vi "Quit.vi"(8 "error in (no error)":errorcluster, 11 "Axis in":refnum<class "Axis.lvclass">) -> (0 "error out":errorcluster)   [LabVIEW 2020, in "Axis.lvclass"]
uses:
  Axis.lvclass
  C:/Users/Jonathan/Documents/Clearpath SDK/CSharp Examples/CLRWrapper/x64/Debug/CLRWrapper.dll
  CSharp Examples/CLRWrapper/x64/Debug/CLRWrapper.dll
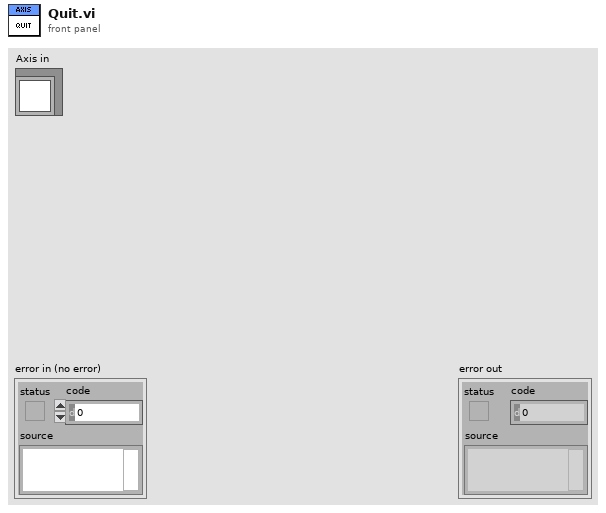
[diagram p1: front panel]
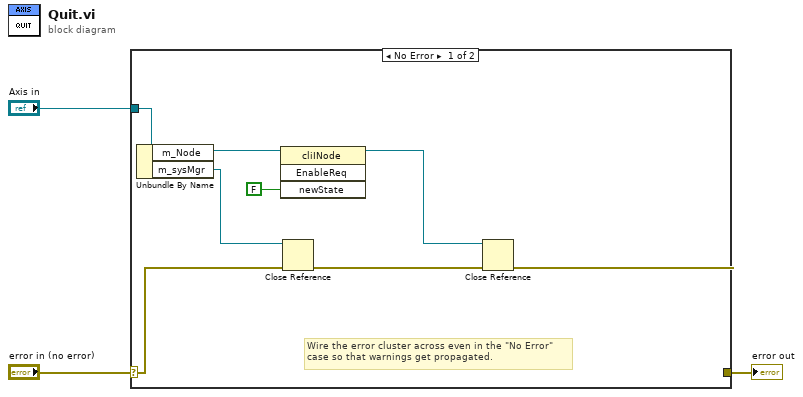
[diagram p0: block diagram]
diagram:
  n1 = case shown="No Error" "error in (no error)" {
    selector: "error in (no error)" -> [w8 w12]
    tunnel: [w4 w12] -> w2
    tunnel: "Axis in" -> [w10 w11]
    frame No Error {
      # "Wire the error cluster across even in the \"No Error\"\ncase so that warnings get propagated."
      n2 = Unbundle By Name(w10) -> ("m_Node"=w6:refnum<k24>, "m_sysMgr"=w9:refnum<k24>)
      n3 = invoke class="cliINode" method="EnableReq"(reference=w6, "newState"=FALSE) -> (reference out=w5:refnum<k24>)  [unwired: 2 in, 3 out]
      n4 = Close Reference(reference=w9, error in (no error)=w8) -> (error out=w4:errorcluster)
      n5 = Close Reference(reference=w5, error in (no error)=w4) -> ()  [unwired: 1 out]
    }
    frame Error {
    }
  }
  "error out" <- w2
